vi "Open Device.vi"(8 "error in (no error)":errorcluster, 9 "Serial Number":string, 10 "Config File":path, 11 "Abstract Topas in":refnum<class "Abstract Topas.lvclass">) -> (0 "error out":errorcluster, 3 "Abstract Topas out":refnum<class "Abstract Topas.lvclass">)   [LabVIEW 2020, in "Abstract Topas.lvclass"]
uses:
  Abstract Topas.lvclass
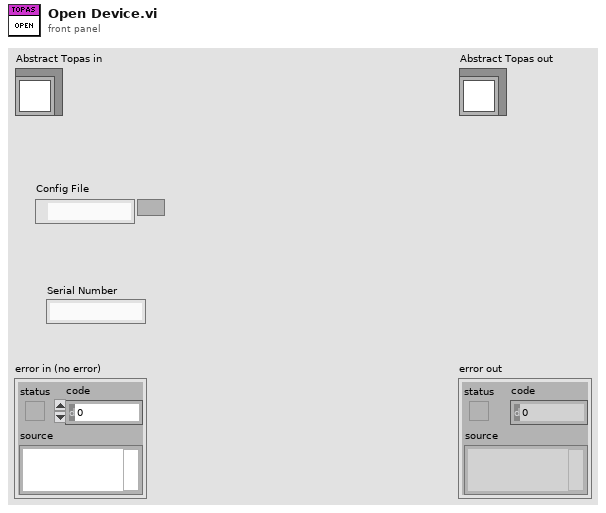
[diagram p1: front panel]
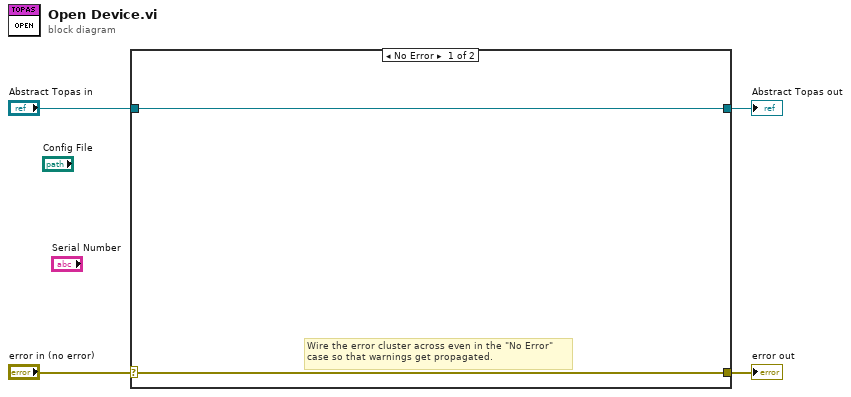
[diagram p0: block diagram]
diagram:
  n1 = case shown="No Error" "error in (no error)" {
    selector: "error in (no error)" -> [w5 w8]
    tunnel: [w5 w8] -> w3
    tunnel: [w6 w7] -> w1
    tunnel: "Abstract Topas in" -> [w6 w7]
    frame No Error {
      # "Wire the error cluster across even in the \"No Error\"\ncase so that warnings get propagated."
    }
    frame Error {
    }
  }
  "error out" <- w3
  "Abstract Topas out" <- w1
